vi "DAQ.setstate.vi"(8 "error in (no error)":errorcluster, 10 "setState":T1, 11 "Instrument.DAQ":refnum<class "Instrument.DAQ.lvclass">) -> (0 "error out":errorcluster, 3 "Instrument.DAQ out":refnum<class "Instrument.DAQ.lvclass">)   [LabVIEW 2019, in "Instrument.Lockin.lvlib" / "Instrument.DAQ.lvclass"]
doc: "---------------------------------------------------------------\nJKI State Machine Objects™\nhttp://jki.net/state-machine-objects/\nCopyright (C) 2005-2015, JKI <info@jki.net>\nALL RIGHTS RESERVEDJKI State Machine Objects (SMO) 1.0.0.4\nJKI - JKI\nCopyright (c) 2015, JKI"
uses:
  Instrument.DAQ.lvclass
  Typedefs/State--enum.ctl
  Instrument.DAQ.lvclass/Instrument.DAQ.ctl
panel:
  # "For instructions on how to use the JKI State Machine Objects, examples and video tutorials, visit:\nhttp://jki.net/state-machine-objects/\n\nJKI State Machine Objects™\nhttp://jki.net/state-machine-objects/\nCopyright (C) 2005-2015, JKI <info@jki.net>\nALL RIGHTS RESERVED"
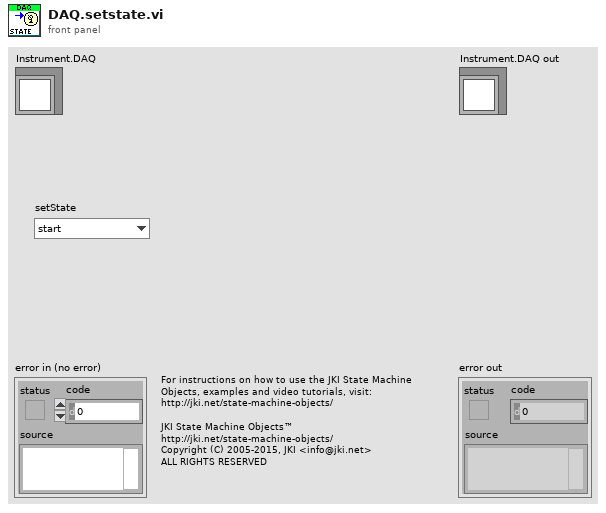
[diagram p1: front panel]
types:
  T1 = typedef "Instrument.Lockin.lvlib/Instrument.DAQ.lvclass/State--enum.ctl" = enum16{"start", "stop", "reset", "start sweep", "stop sweep"}
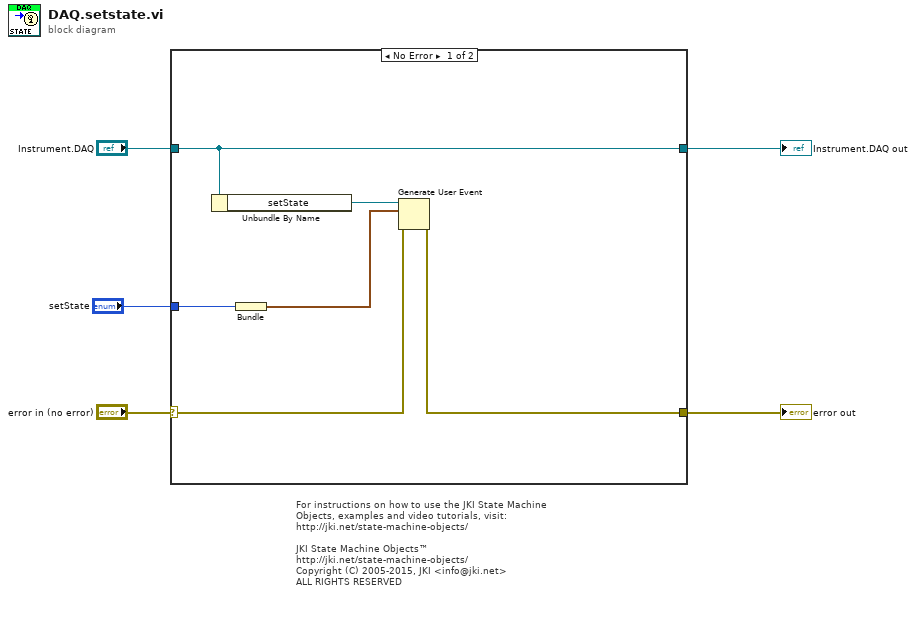
[diagram p0: block diagram]
diagram:
  # "For instructions on how to use the JKI State Machine Objects, examples and video tutorials, visit:\nhttp://jki.net/state-machine-objects/\n\nJKI State Machine Objects™\nhttp://jki.net/state-machine-objects/\nCopyright (C) 2005-2015, JKI <info@jki.net>\nALL RIGHTS RESERVED"
  n1 = case shown="No Error" "error in (no error)" {
    selector: "error in (no error)" -> [w11 w13]
    tunnel: [w9 w13] -> w4
    tunnel: [w8 w12] -> w5
    tunnel: "Instrument.DAQ" -> [w8 w12]
    tunnel: "setState" -> [w6 _]
    frame No Error {
      n2 = Unbundle By Name(w8) -> ("setState"=w10:refnum<user-event>)
      n3 = Bundle("setState"=w6) -> (w7:cluster{"setState":T1})  [unwired: 1 in]
      n4 = Generate User Event(user event=w10, event data cluster=w7, error in=w11) -> (error out=w9:errorcluster)  [unwired: 1 in, 1 out]
    }
    frame Error {
    }
  }
  "error out" <- w4
  "Instrument.DAQ out" <- w5
